vi "Camera.Simulated.DVRToRef.vi"(10 "Ref":T1) -> (2 "Ref":u32 format="%08x")   [LabVIEW 2015, in "Camera.Simulated.lvclass"]
uses:
  Camera.Simulated.lvclass
  PrivateData--Ref.ctl
  PrivateData--Cluster.ctl
  Dependencies--Cluster.ctl
  CircularBuffer/CircularBuffer.lvclass
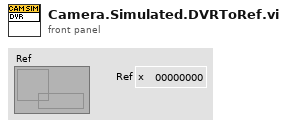
[diagram p1: front panel]
types:
  T1 = typedef "Camera.Simulated.lvclass/PrivateData--Ref.ctl" = refnum<data-value>
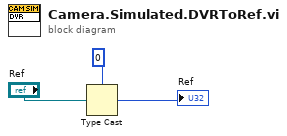
[diagram p0: block diagram]
diagram:
  n1 = Type Cast(type=u32 0 ("Ref"), x="Ref") -> (*(type *) &x=→"Ref":u32)
